vi "GetRawMsg.vi"(8 "error in (no error)":errorcluster, 11 "UpstreamMsgParent in":refnum<class "UpstreamMsgParent.lvclass">) -> (0 "error out":errorcluster, 2 "Msg":string, 3 "UpstreamMsgParent out":refnum<class "UpstreamMsgParent.lvclass">)   [LabVIEW 2020, in "UpstreamMsg.lvlib" / "UpstreamMsgParent.lvclass"]
uses:
  UpstreamMsgParent/UpstreamMsgParent.lvclass
  45e344d1-2595-4bcc-ba58-979c03427db5.vi
  <vilib>/JDP Science/JSONtext/JSONtext.lvlib
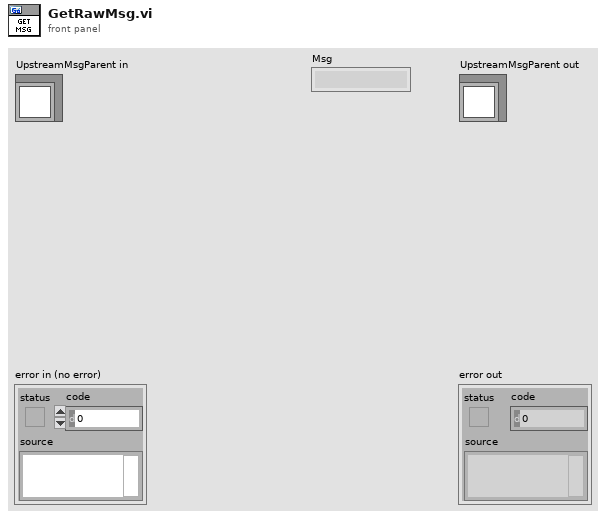
[diagram p1: front panel]
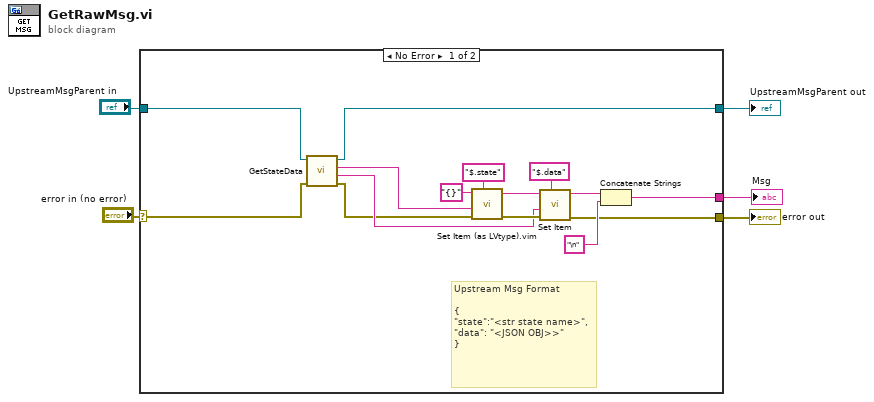
[diagram p0: block diagram]
diagram:
  n1 = case shown="No Error" "error in (no error)" {
    selector: "error in (no error)" -> [w7 w22]
    tunnel: [w13 w22] -> w4
    tunnel: [w10 w21] -> w2
    tunnel: "UpstreamMsgParent in" -> [w11 w21]
    tunnel: [w12 _] -> w1
    frame No Error {
      # "Upstream Msg Format \n\n{\n\"state\":\"<str state name>\",\n\"data\": \"<JSON OBJ>>\"\n}"
      n2 = call-dynamic "GetStateData.vi"("error in (no error)"=w7, "UpstreamMsgParent in"=w11) -> ("error out"=w6:errorcluster, "Data"=w8:string, "State"=w9:string, "UpstreamMsgParent out"=w10:refnum<class "UpstreamMsgParent.lvclass">)  [unwired: 6 in]
      n3 = call "Set Item (as LVtype).vim"("Object (or Item) Path"="$.state", "error in (no error)"=w6, "Anything"=w9, "JSON"="{}") -> ("error out"=w16:errorcluster, "<JSON>"=w18:string)  [unwired: 4 in, 1 out]
      n4 = call <vilib>:"Set Item.vi"("$Path or Item Name"="$.data", "error in (no error)"=w16, "JSON to Insert"=w8, "JSON"=w18) -> ("error out"=w13:errorcluster, "<JSON>"=w15:string)  [unwired: 4 in, 1 out]
      n5 = Concatenate Strings(w15, "\n" ("string")) -> (w12:string)
    }
    frame Error {
    }
  }
  "error out" <- w4
  "UpstreamMsgParent out" <- w2
  "Msg" <- w1
